vi "VeriStand Framework.Create.vi"(8 "error in (no error)":errorcluster, 9 "debug mode (F)":bool, 10 "Engine Data Ref":T1 {"Ptr.End" format="%.0x"; "Ptr.Beg" format="%.0x"}, 11 "Device Item Ref":T2=18446744073709551615 format="%.0x") -> (0 "error out":errorcluster, 3 "VeriStand Framework out":refnum<class "VeriStand DSF.Framework.lvclass">)   [LabVIEW 2017, in "Data Sharing Framework Engine.lvlib" / "VeriStand DSF.Framework.lvclass"]
uses:
  VeriStand DSF.Framework.lvclass
  DSF Core/Built/PharLap x86/Engine/c/DSF.Engine.lvlibp/Engine/Classes/Pointer/DSF.Engine.Pointer.DBL.lvclass
  VeriStand Framework Configuration/VeriStand DSF.Framework.Configuration.lvclass
  Data Sharing Framework Engine.lvlib
  DSF Core/Built/PharLap x86/Engine/c/DSF.Engine.lvlibp/Engine/Classes/Debug/DSF.Engine.Debug Flags.FIFO.lvclass
  DSF Core/Built/PharLap x86/Engine/c/DSF.Engine.lvlibp/Engine/Classes/Debug/DSF.Engine.Debug Flags.lvclass
  <vilib>/NI Veristand/Custom Device API/Custom Device Item Ref.ctl
  <vilib>/NI VeriStand/Custom Device API/Custom Device API.lvlib
  <vilib>/NI Veristand/Custom Device API/Data Table Ref.ctl
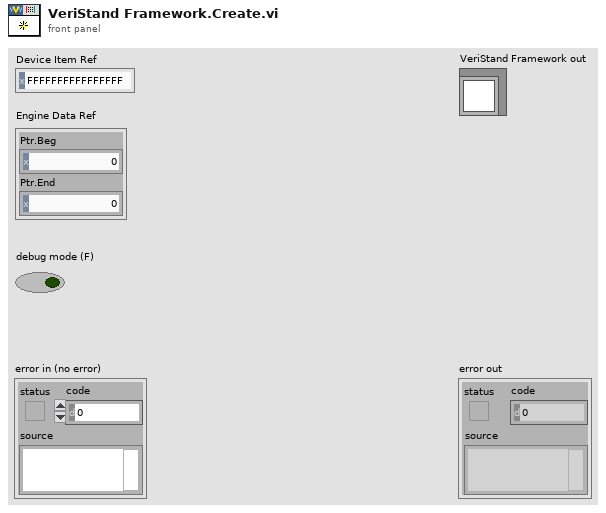
[diagram p1: front panel]
types:
  T1 = typedef "Custom Device API.lvlib/Data Table Ref.ctl" = cluster{"Ptr.Beg":u64, "Ptr.End":u64}
  T2 = typedef "Custom Device API.lvlib/Custom Device Item Ref.ctl" = u64
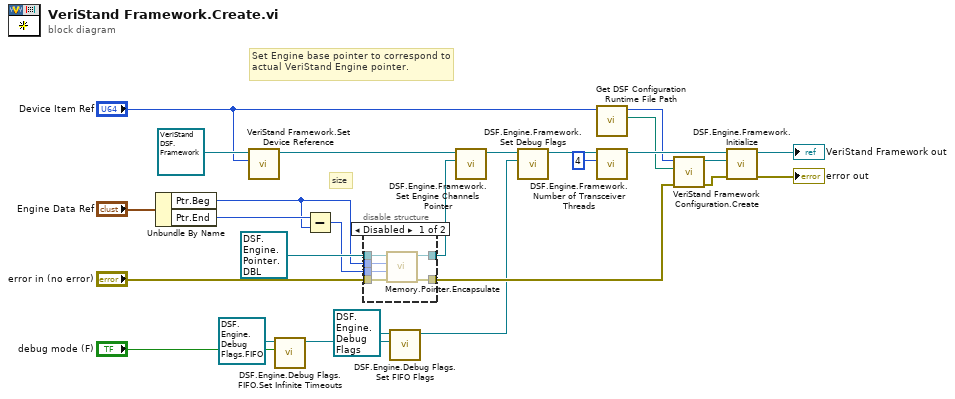
[diagram p0: block diagram]
diagram:
  # "size"
  # "Set Engine base pointer to correspond to actual VeriStand Engine pointer."
  n1 = Unbundle By Name("Engine Data Ref") -> ("Ptr.Beg"=w21:u64, "Ptr.End"=w23:u64)
  n2 = call "VeriStand Framework.Set Device Reference.vi"("Device Item Ref"="Device Item Ref", "VeriStand Framework in"=refnum<class "VeriStand DSF.Framework.lvclass"> refnum) -> ("VeriStand Framework out"=w24:refnum<class "VeriStand DSF.Framework.lvclass">)  [unwired: 9 in]
  n3 = call "DSF.Engine.Debug Flags.FIFO.Set Infinite Timeouts.vi"("infinite timeouts"="debug mode (F)", "FIFO Debug Flags in"=refnum<class "DSF.Engine.Debug Flags.FIFO.lvclass"> refnum) -> ("FIFO Debug Flags out"=w8:refnum<class "DSF.Engine.Debug Flags.FIFO.lvclass">)  [unwired: 9 in]
  n4 = Subtract(x=w23, y=w21) -> (x-y=w22:u64)
  n5 = disable-structure shown="Disabled" {
    disable-tunnel: refnum<class "DSF.Engine.Pointer.DBL.lvclass"> refnum ("Engine Channels Pointer") -> [w32 w34]
    disable-tunnel: w22 -> [w31 _]
    disable-tunnel: w21 -> [w30 _]
    disable-tunnel: "error in (no error)" -> [w29 w33]
    disable-tunnel: [w28 w33] -> w9
    disable-tunnel: [w27 w34] -> w15
    frame Disabled {
      n6 = call "Memory.Pointer.Encapsulate.vi"("error in (no error)"=w29, "size"=w31, "address"=w30, "Pointer type"=w32) -> ("error out"=w28:errorcluster, "Pointer out"=w27:refnum<class "DSF.Engine.Pointer.DBL.lvclass">)  [unwired: 6 in]
    }
    frame Enabled {
    }
  }
  n7 = call "DSF.Engine.Debug Flags.Set FIFO Flags.vi"("FIFO"=w8, "Debug Flags in"=refnum<class "DSF.Engine.Debug Flags.lvclass"> refnum) -> ("Debug Flags out"=w3:refnum<class "DSF.Engine.Debug Flags.lvclass">)  [unwired: 9 in]
  n8 = call "DSF.Engine.Framework.Set Engine Channels Pointer.vi"("Engine Channels Pointer"=w15, "Framework in"=w24) -> ("Framework out"=w5:refnum<class "VeriStand DSF.Framework.lvclass">)  [unwired: 9 in]
  n9 = call "DSF.Engine.Framework.Set Debug Flags.vi"("Debug Flags"=w3, "Framework in"=w5) -> ("Framework out"=w4:refnum<class "VeriStand DSF.Framework.lvclass">)  [unwired: 9 in]
  n10 = call "Get DSF Configuration Runtime File Path.vi"("Item Ref in"="Device Item Ref") -> ("Path"=w12:path, "Item Ref out"=w11:T2)  [unwired: 7 in, 2 out]
  n11 = call "DSF.Engine.Framework.Number of Transceiver Threads.vi"("transceiver count"=4, "Framework in"=w4) -> ("Framework out"=w14:refnum<class "VeriStand DSF.Framework.lvclass">)  [unwired: 8 in, 1 out]
  n12 = call "VeriStand Framework Configuration.Create.vi"("error in (no error)"=w9, "configuration path"=w12, "Device Item Ref"=w11) -> ("error out"=w10:errorcluster, "VeriStand Framework Configuration"=w17:refnum<class "VeriStand DSF.Framework.Configuration.lvclass">)  [unwired: 7 in]
  n13 = call "DSF.Engine.Framework.Initialize.vi"("error in (no error)"=w10, "Framework Configuration"=w17, "Framework type"=w14) -> ("error out"=→"error out":errorcluster, "Framework out"=→"VeriStand Framework out":refnum<class "VeriStand DSF.Framework.lvclass">)  [unwired: 7 in]
